vi "Example Callback - Random Range.vi"(8 "max":i32, 11 "min":i32) -> (3 "random":i32)   [LabVIEW 2010]
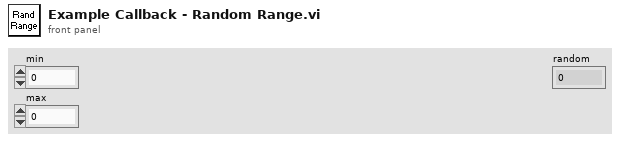
[diagram p1: front panel]
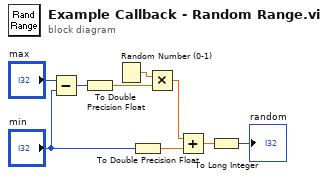
[diagram p0: block diagram]
diagram:
  n1 = Subtract(x="max", y="min") -> (x-y=w5:i32)
  n2 = To Double Precision Float(number=w5) -> (double precision float=w4:dbl)
  n3 = Random Number (0-1)() -> (number: 0 to 1=w8:dbl)
  n4 = To Double Precision Float(number="min") -> (double precision float=w3:dbl)
  n5 = Multiply(x=w8, y=w4) -> (x*y=w9:dbl)
  n6 = Add(x=w9, y=w3) -> (x+y=w7:dbl)
  n7 = To Long Integer(number=w7) -> (32bit integer=→"random":i32)
